vi "destroy.vi"(8 "error in":errorcluster, 11 "stream publisher in":refnum<class "data bus stream subscriber.lvclass">) -> (0 "error out":errorcluster)   [LabVIEW 2013, in "data bus stream subscriber.lvclass"]
uses:
  data bus stream subscriber.lvclass
  data bus stream subscriber.lvclass/data bus stream subscriber.ctl
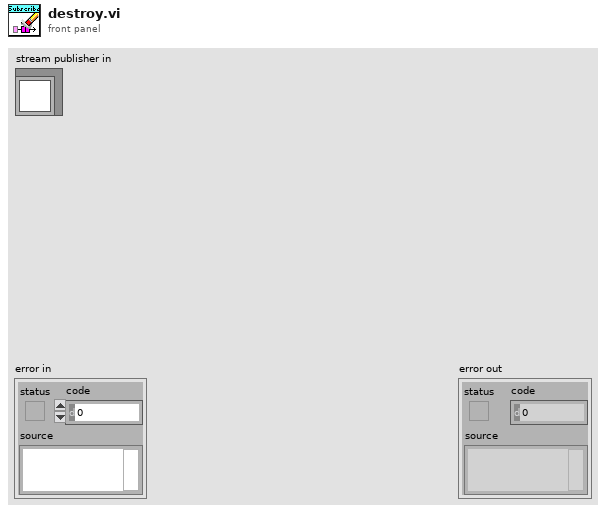
[diagram p1: front panel]
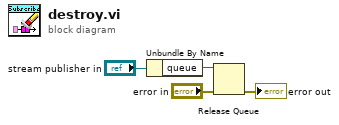
[diagram p0: block diagram]
diagram:
  n1 = Unbundle By Name("stream publisher in") -> ("queue"=w1:refnum<queue>)
  n2 = Release Queue(queue=w1, error in (no error)="error in") -> (error out=→"error out":errorcluster)  [unwired: 1 in, 2 out]
